vi "CIET Data Client.vi"() -> ()   [LabVIEW 2017]
uses:
  <vilib>/OPCUA/controls/Write Status.ctl
  <vilib>/OPCUA/controls/NodeId.ctl
  <vilib>/OPCUA/client/Multiple Write Double Array.vi
  <vilib>/OPCUA/NI OPC UA Client.lvlib
panel:
  out "CIET Readings":dbl[](array[numeric])
  in  "Stop Reading":bool
  out "Log Loop":i32
  in  "Stop Control":bool
  out "Send Loop":i32
  in  "Time Stamp":timestamp
  in  "Node Status":T1 items=["Good"=0, "Uncertain_InitialValue"=1083310080, "Uncertain_LastUsableValue"=1083179008, "Uncertain_SensorNotAccurate"=1083375616, "Uncertain_EngineeringUnitsExceeded"=1083441152, "Bad_NoCommunication"=2150694912, "Bad_NotReadable"=2151284736, "Bad_NotWritable"=2151350272, "Bad_OutOfRange"=2151415808, "Bad_WaitingForInitialData"=2150760448]
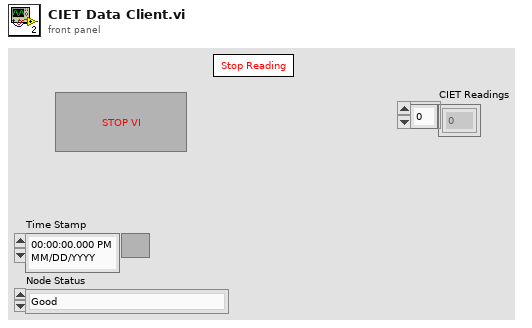
[diagram p1: front panel]
types:
  T1 = typedef "Write Status.ctl" = u32
  T2 = typedef "OPC UA Client Refnum.ctl" = refnum<k21>
  T3 = typedef "NodeId.ctl" = string
  T4 = cluster{"node ID":T3, "value":dbl[], "timestamp (current time)":timestamp, "node status":T1}
  T5 = cluster{"node ID":T3, "value":dbl[], "timestamp (current time)":timestamp, "node status":T1}[]
  T6 = typedef "Subscription ID.ctl" = u32
  T7 = typedef "Subscription Data Change.ctl" = cluster{"node ID":T3, " value":variant, "timestamp":timestamp, "data type":T8, "status code":T9}
  T8 = typedef "Data Type.ctl" = u16
  T9 = typedef "OPC UA StatusCode.ctl" = u32
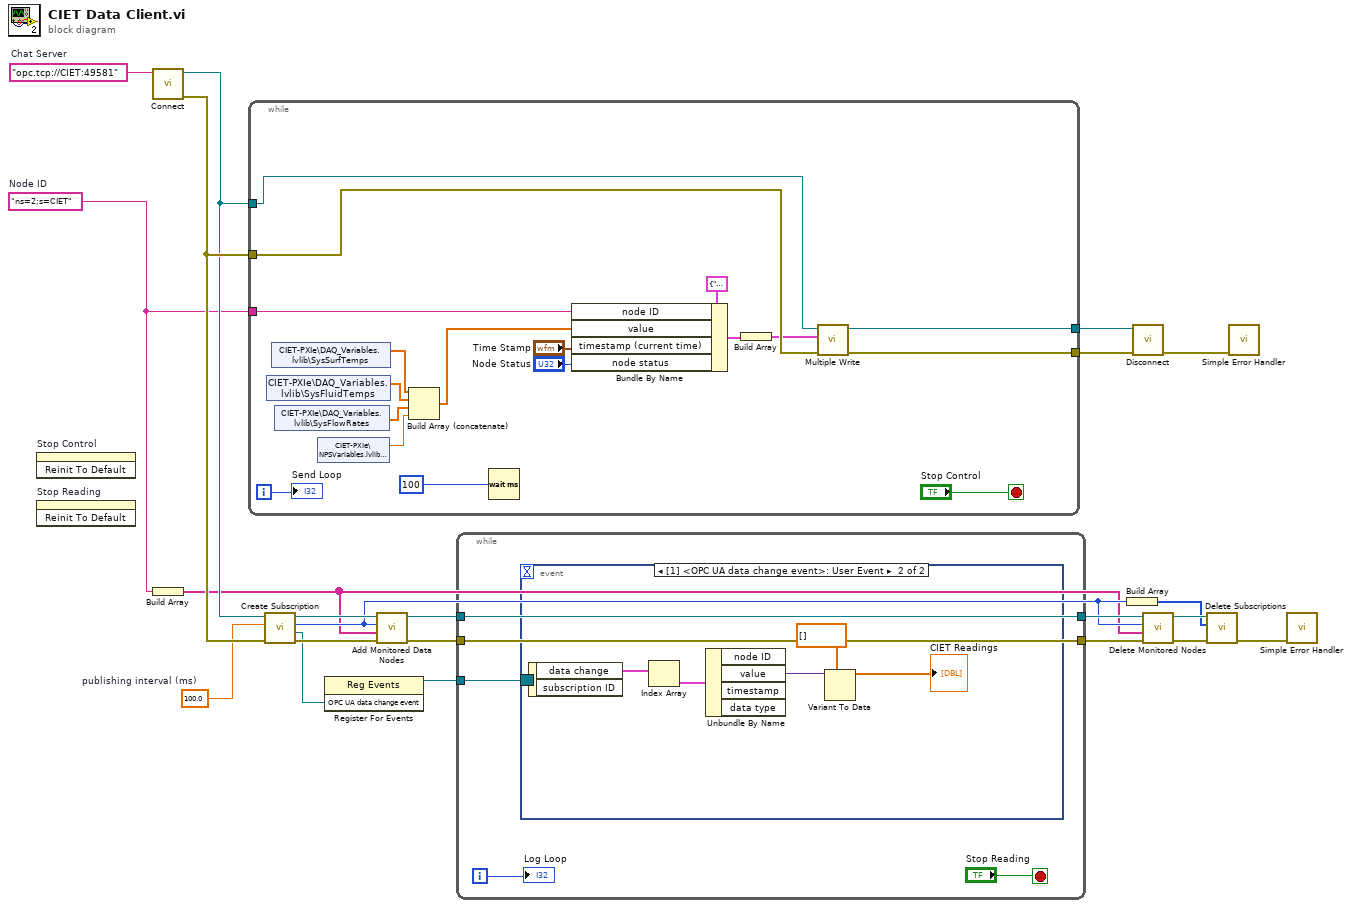
[diagram p0: block diagram]
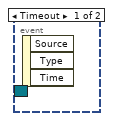
[diagram p2: hidden frame]
diagram:
  w1 = 100.0  # publishing interval (ms)
  w5 = "ns=2;s=CIET"  # Node ID
  w21 = "opc.tcp://CIET:49581"  # Chat Server
  n1 = invoke on="Stop Control" class="Bool (strict)" method="Reinit To Default"() -> ()  [unwired: 3 in, 3 out]
  n2 = invoke on="Stop Reading" class="Bool (strict)" method="Reinit To Default"() -> ()  [unwired: 3 in, 3 out]
  n3 = call <vilib>:"Connect.vi"("server endpoint URL"=w21) -> ("error out"=w20:errorcluster, "OPC UA client refnum out"=w19:T2)  [unwired: 8 in, 1 out]
  n4 = Build Array(w5) -> (w4:string[])
  n5 = while {
    tunnel: w5 -> [w38]
    tunnel: w19 -> [w35]
    tunnel: w20 -> [w34]
    tunnel: [w37] -> w3
    tunnel: [w36] -> w2
    i -> [w39]
    stop <- "Stop Control" stop-if-true
    n6 = shared-variable "CIET-PXIe\\DAQ_Variables.lvlib\\SysFluidTemps"() -> (w28:sgl[])  [unwired: 1 in, 1 out]
    n7 = shared-variable "CIET-PXIe\\DAQ_Variables.lvlib\\SysSurfTemps"() -> (w27:sgl[])  [unwired: 1 in, 1 out]
    n8 = shared-variable "CIET-PXIe\\DAQ_Variables.lvlib\\SysFlowRates"() -> (w29:sgl[])  [unwired: 1 in, 1 out]
    n9 = shared-variable "CIET-PXIe\\NPSVariables.lvlib\\Time"() -> (w30:sgl)  [unwired: 1 in, 1 out]
    n10 = Build Array (concatenate)(w27, w28, w29, w30) -> (w26:sgl[])
    n11 = Wait (ms)(milliseconds to wait=u32 100) -> ()  [unwired: 1 out]
    n12 = Bundle By Name(cluster=T4 {"node ID"="", "value"=[], "timestamp (current time)"=timestamp(0 s since 1904-01-01), "node status"=0} ("request"), "node ID"=w38, "value"=w26, "timestamp (current time)"="Time Stamp", "node status"="Node Status") -> (w24:T4)
    n13 = Build Array(w24) -> (w23:T5)
    n14 = call-poly <vilib>:"Multiple Write.vi"("error in (no error)"=w34, "requests"=w23, "OPC UA client refnum in"=w35) -> ("error out"=w36:errorcluster, "OPC UA client refnum out"=w37:T2)  [unwired: 5 in, 2 out]
    "Send Loop" <- w39
  }
  n15 = call <vilib>:"Create Subscription.vi"("error in (no error)"=w20, "publishing interval (1000 ms)"=w1, "OPC UA client refnum in"=w19) -> ("error out"=w17:errorcluster, "OPC UA data change event"=w16:refnum<user-event>, "subscription ID out"=w8:T6, "OPC UA client refnum out"=w18:T2)  [unwired: 4 in, 1 out]
  n16 = register-events(w16) -> (reference out=w15:refnum<event-registration>)  [unwired: 2 in, 1 out]
  n17 = call <vilib>:"Add Monitored Data Nodes.vi"("error in (no error)"=w17, "node IDs"=w4, "subscription ID in"=w8, "OPC UA client refnum in"=w18) -> ("error out"=w12:errorcluster, "OPC UA client refnum out"=w14:T2)  [unwired: 4 in, 2 out]
  n18 = while {
    tunnel: w15 -> [w45]
    tunnel: w14 -> [w43]
    tunnel: [w43] -> w13
    tunnel: w12 -> [w42]
    tunnel: [w42] -> w11
    i -> [w41]
    stop <- "Stop Reading" stop-if-true
    n19 = event shown="[1] <OPC UA data change event>: User Event" {
      selector: w45 -> [_ _]
      dyn-events: _ -> [_ _]
      timeout: _ -> [_ _]
      event Timeout {
        n20 = event-data() -> ()  [unwired: 1 in, 3 out]
      }
      event User Event {
        n21 = event-data() -> ("data change"=w50:T7[])  [unwired: 1 in, 1 out]
        n22 = Index Array(array=w50) -> (element=w49:T7)  [unwired: 1 in]
        n23 = Unbundle By Name(w49) -> ("value"=w48:variant)  [unwired: 3 out]
        n24 = Variant To Data(type=dbl[] [], Variant=w48) -> (data=→"CIET Readings":dbl[])  [unwired: 1 in, 1 out]
      }
    }
    "Log Loop" <- w41
  }
  n25 = Build Array(w8) -> (w7:T6[])
  n26 = call <vilib>:"Disconnect.vi"("error in (no error)"=w2, "OPC UA client refnum in"=w3) -> ("error out"=w22:errorcluster)  [unwired: 9 in]
  n27 = call <vilib>:"Delete Monitored Nodes.vi"("error in (no error)"=w11, "node IDs"=w4, "subscription ID in"=w8, "OPC UA client refnum in"=w13) -> ("error out"=w9:errorcluster, "OPC UA client refnum out"=w10:T2)  [unwired: 3 in, 3 out]
  n28 = call <vilib>:"Delete Subscriptions.vi"("error in (no error)"=w9, "subscription IDs"=w7, "OPC UA client refnum in"=w10) -> ("error out"=w6:errorcluster)  [unwired: 6 in, 2 out]
  n29 = call <vilib>:"Simple Error Handler.vi"("error in (no error)"=w22) -> ()  [unwired: 4 in, 5 out]
  n30 = call <vilib>:"Simple Error Handler.vi"("error in (no error)"=w6) -> ()  [unwired: 4 in, 5 out]
